vi "3D_Traverse_move.vi"(0 "Mode":T3=enum."Read traverse position", 1 "Route Checking?":bool=TRUE, 2 "Row Number":i32=-1, 5 "Position":dbl[](array[numeric])=[0.0, 0.0, 0.0] format="%#.2f", 7 "Work in Tunnel Coordinates":T1, 11 "Simulate/Run":T2=enum."Run VI", 12 "Traverse name":string, 13 "Backlash Compensation?":bool=TRUE, 14 "Currently on Point":i32=-1) -> (3 "Model  Roll        Pitch       Yaw (deg)":dbl[](array[numeric]) format="%#.2f", 4 "Trav Position achieved":dbl[](array[numeric]) format="%#.2f", 15 "Error String":string)   [LabVIEW 2011]
uses:
  Trav_mode.ctl
  Controls/User_Specific_mode.ctl
  Controls/Tunnel_Coordinates.ctl
  Controls/Global_mode.ctl
  Route mapping/Route_Display_Mode.ctl
  ADAM Client/Sub VIs/ADAM Controls/Update_scan_value.ctl
  Controls/In_Range.ctl
  Globals/Trav_pos_global.vi
  Globals/Constants_global.vi
  Route mapping/Route_mapping_global.vi
panel:
  in  "Position Increment":dbl[](array[numeric])=[0.0, 0.0, 0.0] step=0.1 format="%#.2f"
  out "Traverses Available":string[](array[string])
  in  "Traverse":u16(ring) items=["A_Tunnel", "Aero_Enclosure", "Aero_Sting", "Aero_ThroughWall", "Aero_Tunnel", "Angle_Calibrator", "B_Tunnel", "D_Tunnel", "Dummy_Traverse", "EnFlo_Stack", "EnFlo_Tunnel", "EnFlo_Turntable", "Laser_Meas_Traverse", "Pitch_Yaw", "PIV_Traverse", "Tank"]
  # "X                Y                   Z"
  # "X                Y                   Z"
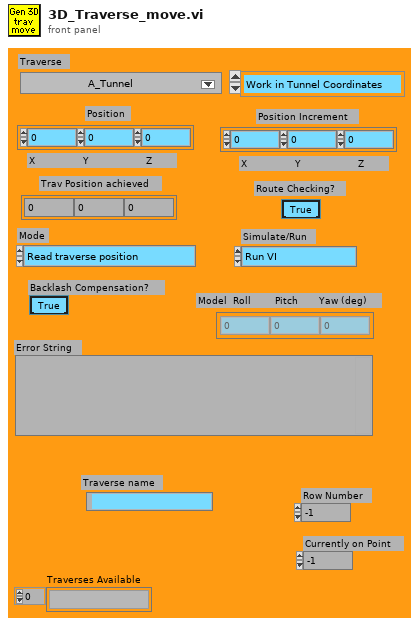
[diagram p1: front panel]
types:
  T1 = typedef "Tunnel_Coordinates.ctl" = enum16{"Work in Tunnel Coordinates", "Work in Model Coordinates"}
  T2 = typedef "User_Specific_mode.ctl" = enum16{"Check VI only", "Run VI"}
  T3 = typedef "Trav_mode.ctl" = enum16{"Move traverse", "Read traverse position", "Teach Position"}
  T4 = typedef "Global_mode.ctl" = enum16{"Read Global", "Load Global From File", "Write Global to File"}
  T5 = enum16{"To Traverse Coordinates", "To User Coordinates"}
  T6 = typedef "Route_Display_Mode.ctl" = enum16{"Display View Always", "Display View on Crash"}
  T7 = typedef "Update_scan_value.ctl" = cluster{"Channel Name":string, "New Value":dbl}
  T8 = typedef "In_Range.ctl" = enum16{"%", "±", "% & ±"}
  T9 = typedef "Box_size.ctl" = cluster{"Max":dbl, "Min":dbl}[]
  T10 = typedef "Exclude_cluster.ctl" = cluster{"Sizes":T9, "Name":string, "Exclude Type":T11}
  T11 = typedef "Exclusion_type.ctl" = enum16{"Exclude completely", "Allow only vertical moves"}
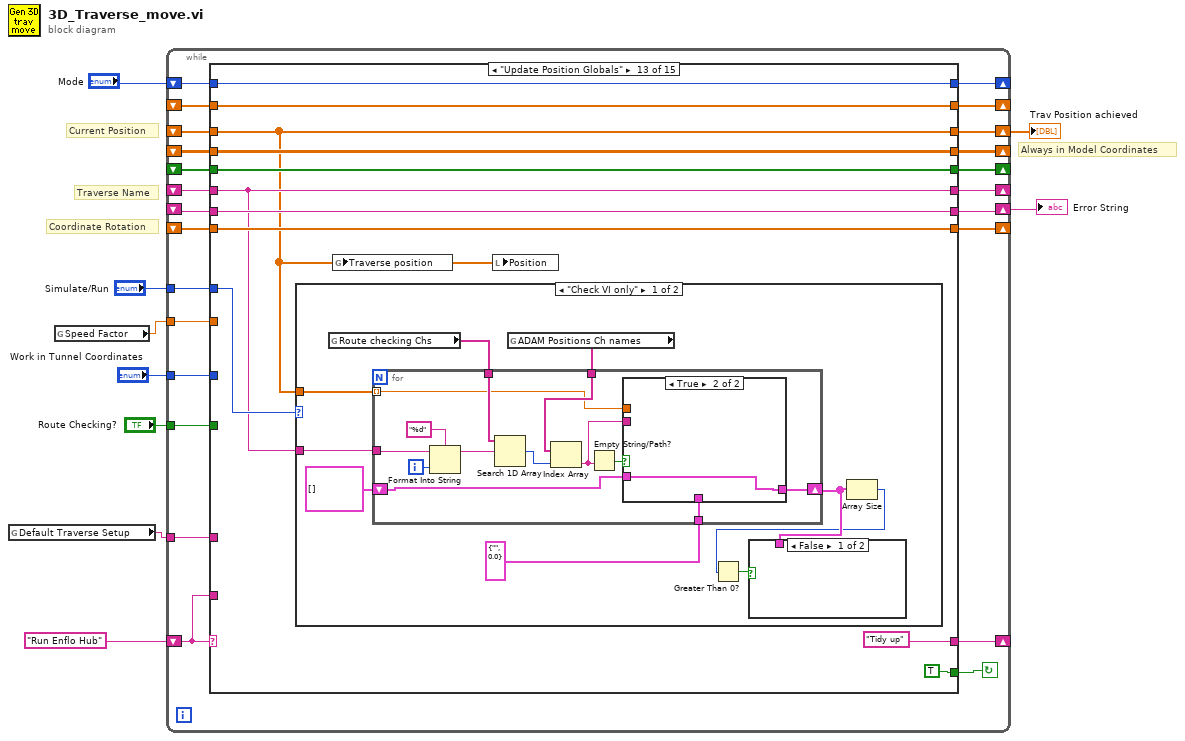
[diagram p0: block diagram]
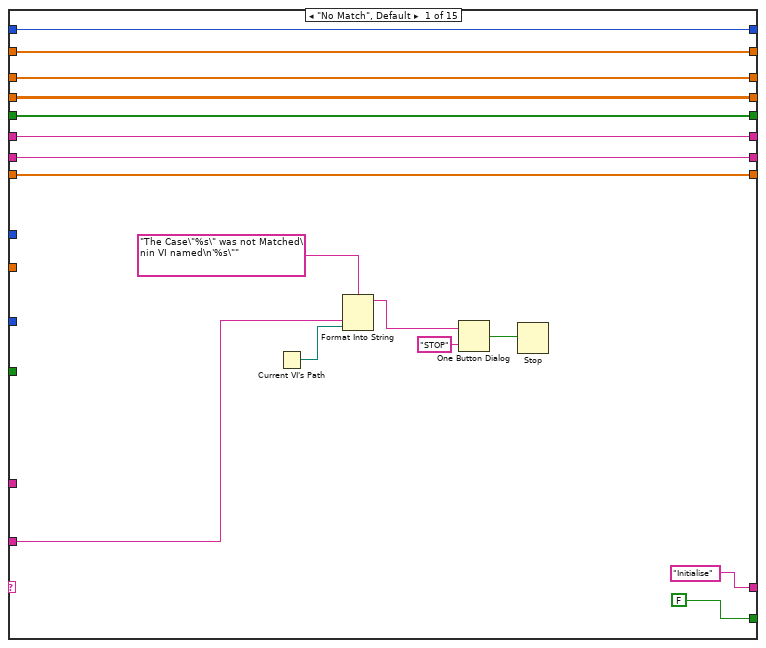
[diagram p2: hidden frame]
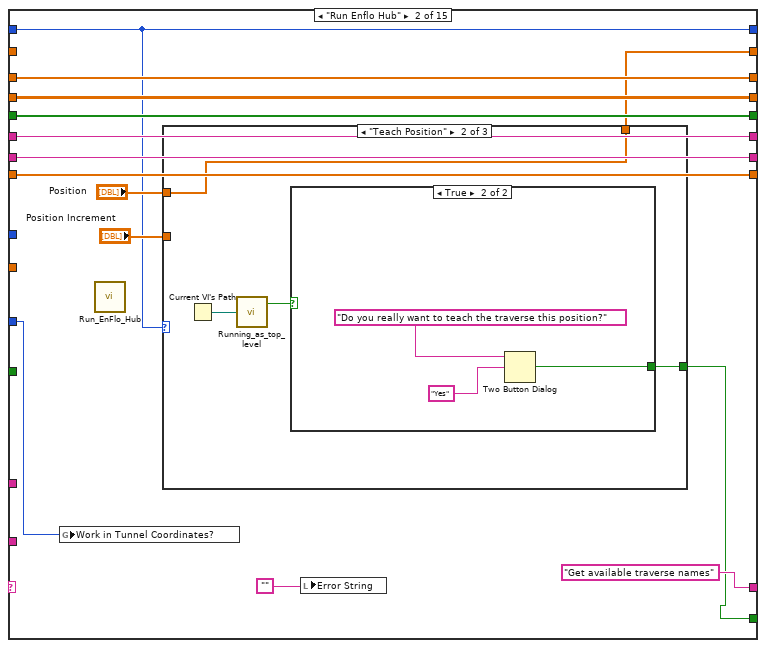
[diagram p3: hidden frame]
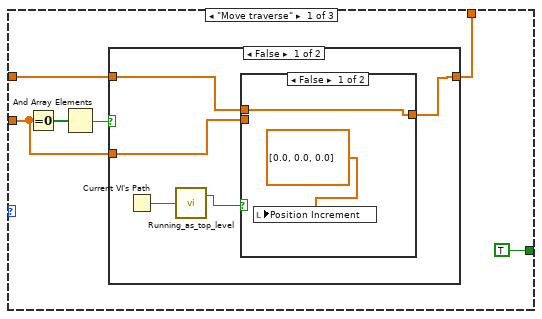
[diagram p4: hidden frame]
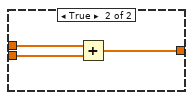
[diagram p5: hidden frame]
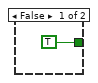
[diagram p7: hidden frame]
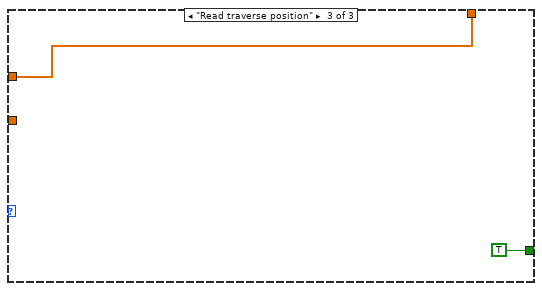
[diagram p8: hidden frame]
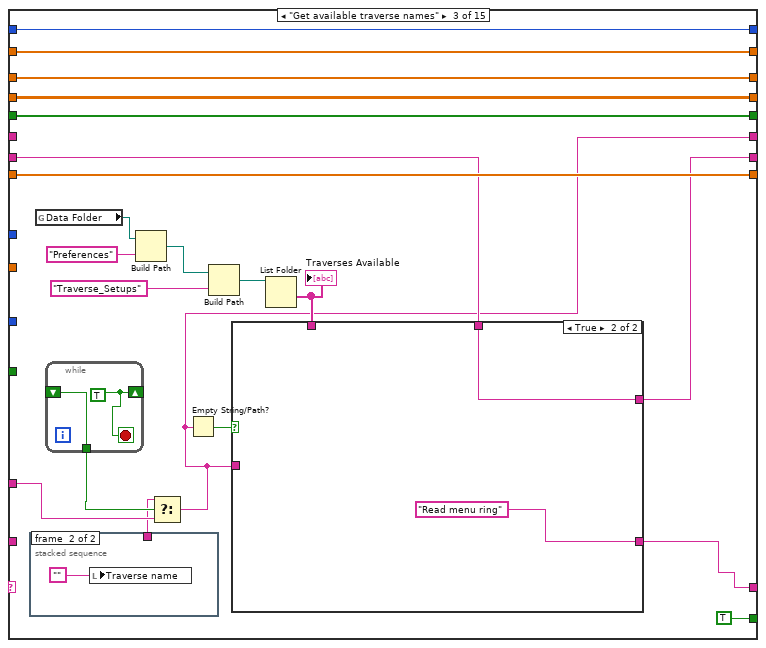
[diagram p9: hidden frame]
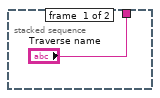
[diagram p10: hidden frame]
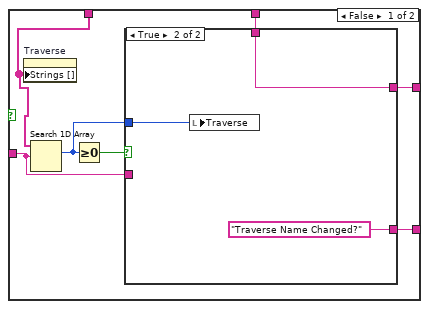
[diagram p11: hidden frame]
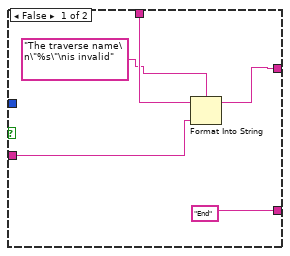
[diagram p12: hidden frame]
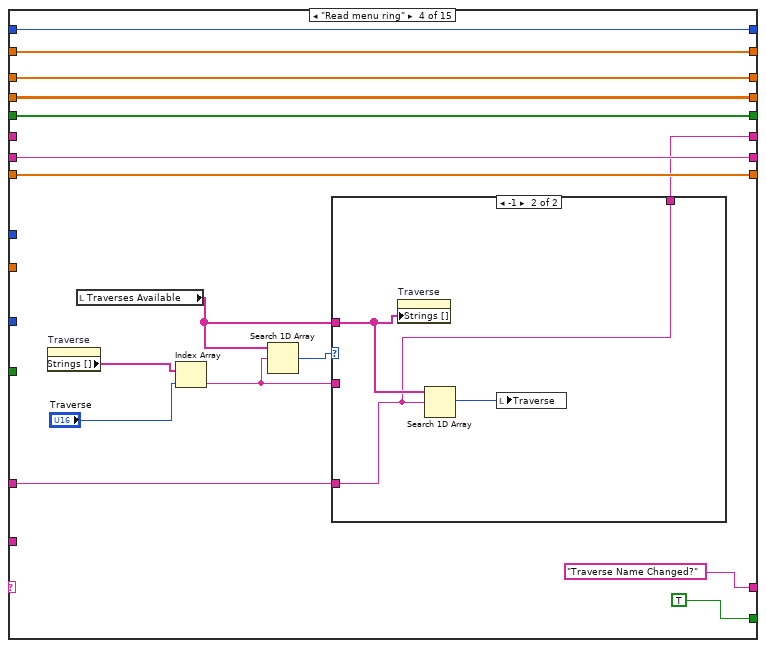
[diagram p13: hidden frame]
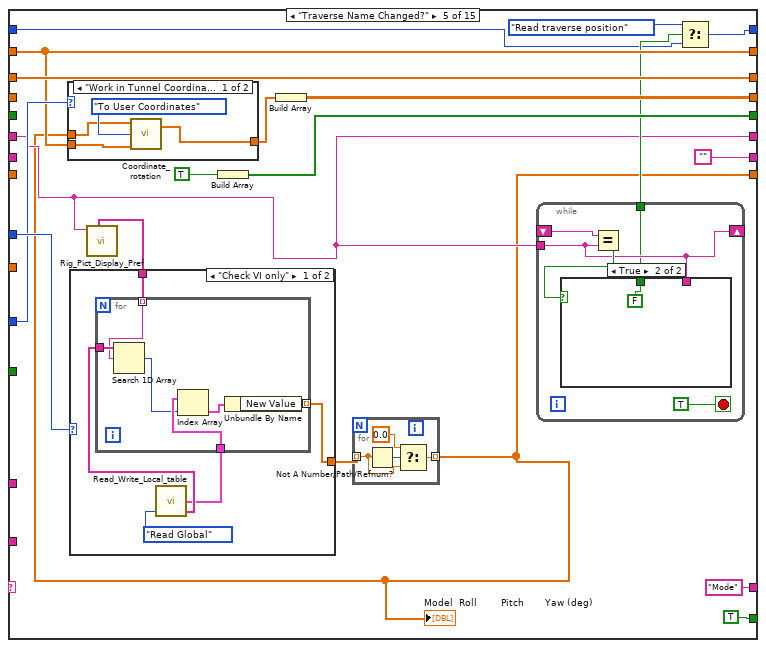
[diagram p15: hidden frame]
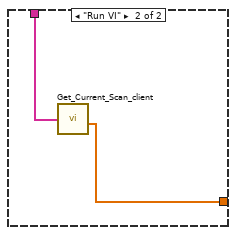
[diagram p16: hidden frame]
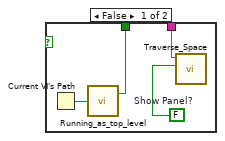
[diagram p18: hidden frame]
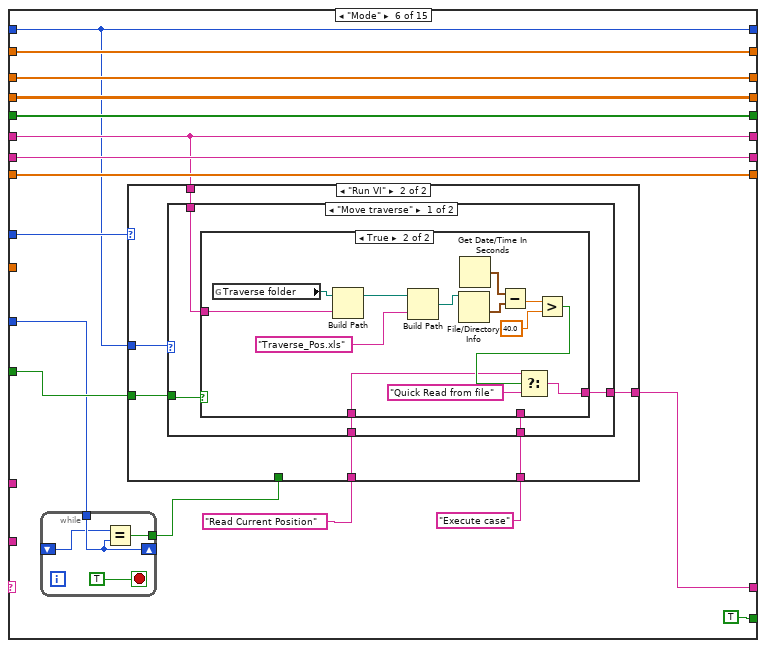
[diagram p19: hidden frame]
diagram:
  # "Always in Model Coordinates"
  # "Current Position"
  # "Coordinate Rotation"
  # "Traverse Name"
  n1 = global read "Trav_pos_global.vi" "Default Traverse Setup"() -> (w2:string)
  n2 = global read "Trav_pos_global.vi" "Speed Factor"() -> (w6:dbl)
  n3 = while {
    shift-left: "Run Enflo Hub" -> [w31]
    shift-right: [w32] -> _
    shift-right: [w29] -> _
    shift-left: _ -> [w27]
    tunnel: "Simulate/Run" -> [w30]
    shift-right: [w28] -> w7
    shift-left: _ -> [w26]
    shift-right: [w24] -> _
    shift-left: _ -> [w25]
    shift-right: [w19] -> _
    shift-left: _ -> [w18]
    shift-right: [w21] -> _
    shift-left: _ -> [w20]
    shift-right: [w22] -> w3
    shift-left: _ -> [w23]
    tunnel: w6 -> [w17]
    tunnel: "Work in Tunnel Coordinates" -> [w16]
    tunnel: "Route Checking?" -> [w15]
    tunnel: w2 -> [w14]
    shift-right: [w13] -> _
    shift-left: _ -> [w12]
    shift-right: [w10] -> _
    shift-left: "Mode" -> [w11]
    stop <- w33 continue-if-true
    n4 = case shown="\"Update Position Globals\"" w31 {
      tunnel: [FALSE w55 TRUE TRUE TRUE TRUE w264 TRUE ("T button?") TRUE w352 w381 TRUE TRUE TRUE FALSE] -> w33
      tunnel: ["Initialise" "Get available traverse names" w101 "Traverse Name Changed?" "Mode" w213 w253 "Perform Route Check" w314 "Display Traverse Views" w388 "Update Position Globals" "Tidy up" "End" "End"] -> w32
      tunnel: w31 -> [w44 _ _ _ _ _ _ _ _ _ _ _ _ _ _]
      tunnel: w30 -> [_ _ _ _ w163 w214 w258 _ w310 _ w386 _ w454 _ w544]
      tunnel: [w41 w62 w94 w133 w156 w205 w266 w290 w309 w358 w393 w429 w453 w496 w540] -> w29
      tunnel: [w40 w61 w99 w146 "" w215 w265 "" w319 w349 w390 w418 w458 w498 w547] -> w28
      tunnel: w27 -> [w41 w62 _ _ w156 w205 w266 w290 w309 w358 w393 w429 w453 w496 w540]
      tunnel: w26 -> [w40 w61 w98 w146 _ w215 _ _ _ w350 w390 _ w458 w499 w547]
      tunnel: w25 -> [w39 w60 w111 w145 _ w216 w262 w293 w305 w345 w397 w425 w457 w502 w541]
      tunnel: [w39 w60 w111 w145 w153 w216 w262 w293 w305 w345 w397 w425 w457 w502 w541] -> w24
      tunnel: w23 -> [w38 w59 w110 w144 w167 w207 w259 _ w317 w357 w396 _ w452 w500 w542]
      tunnel: [w38 w59 w110 w144 w167 w207 w260 w292 w318 w357 w396 w423 w452 w500 w542] -> w22
      tunnel: [w37 w58 w109 w143 w168 w218 w268 w297 w316 w356 w394 w427 w459 w503 w548] -> w21
      tunnel: w20 -> [w37 w58 w109 w143 _ w218 w268 w297 _ w356 w394 w427 w459 w503 w548]
      tunnel: [w36 w57 w108 w142 w165 w217 w267 w296 w321 w355 w395 w421 w460 w504 w549] -> w19
      tunnel: w18 -> [w36 w57 w108 w142 _ w217 w267 w296 _ w355 w395 w421 w460 w504 w549]
      tunnel: w17 -> [_ _ _ _ _ _ _ _ _ _ _ w428 _ _ _]
      tunnel: w16 -> [_ w54 _ _ w162 w209 w263 w294 w327 w346 _ w426 _ _ w543]
      tunnel: w15 -> [_ _ _ _ _ w210 _ _ _ _ _ w417 _ _ _]
      tunnel: w14 -> [_ _ w95 w137 _ _ _ _ _ _ _ _ _ _ _]
      tunnel: [w35 w53 w92 w135 w161 w206 w252 w291 w304 w348 w380 w416 w456 w495 w545] -> w13
      tunnel: w12 -> [w35 _ w92 w135 w161 w206 w252 w291 w304 w348 w380 w416 w456 w495 w545]
      tunnel: w11 -> [w34 w50 w91 w134 w157 w204 w251 w286 w303 w347 w379 w415 w455 w494 w539]
      tunnel: [w34 w50 w91 w134 w158 w204 w251 w286 w303 w347 w379 w415 w455 w494 w539] -> w10
      frame "No Match", Default {
        n5 = Current VI's Path() -> (path=w43:path)
        n6 = Format Into String(format string="The Case\"%s\" was not Matched\nin VI named\n'%s\"" ("Format String"), w44, w43) -> (resulting string=w47:string)  [unwired: 2 in, 1 out]
        n7 = One Button Dialog(message=w47, button name ("OK")="STOP") -> (true=w45:bool)
        n8 = Stop(stop? (T)=w45) -> ()
      }
      frame "Run Enflo Hub" {
        n9 = global write "Trav_pos_global.vi" "Work in Tunnel Coordinates?"(w54) -> ()
        n10 = call "Run_EnFlo_Hub.vi"() -> ()  [unwired: 8 out]
        n11 = case shown="\"Teach Position\"" w50 {
          tunnel: [TRUE ("T button?") w82 TRUE ("T button?")] -> w55
          tunnel: [w66 w81 w90] -> w53
          tunnel: "Position" -> [w65 w81 w90]
          tunnel: "Position Increment" -> [w64 _ _]
          frame "Move traverse" {
            n12 = Equal To 0?(x=w64) -> (x = 0?=w68:bool[])
            n13 = And Array Elements(Boolean array=w68) -> (logical AND=w67:bool)
            n14 = case shown="False" w67 {
              tunnel: [w70 w80] -> w66
              tunnel: w65 -> [w72 w80]
              tunnel: w64 -> [w71 _]
              frame False {
                n15 = Current VI's Path() -> (path=w74:path)
                n16 = call "Running_as_top_level.vi"("Vi path name"=w74) -> ("Top Level"=w73:bool)  [unwired: 1 out]
                n17 = case shown="False" w73 {
                  tunnel: w72 -> [w76 w79]
                  tunnel: w71 -> [_ w78]
                  tunnel: [w76 w77] -> w70
                  frame False {
                    n18 = local write "Position Increment"(dbl[] [0.0, 0.0, 0.0] ("Position Increment")) -> ()
                  }
                  frame True {
                    n19 = Add(x=w79, y=w78) -> (x+y=w77:dbl[])
                  }
                }
              }
              frame True {
              }
            }
          }
          frame "Teach Position" {
            n20 = Current VI's Path() -> (path=w84:path)
            n21 = call "Running_as_top_level.vi"("Vi path name"=w84) -> ("Top Level"=w83:bool)  [unwired: 1 out]
            n22 = case shown="True" w83 {
              tunnel: [TRUE ("T button?") w86] -> w82
              frame False {
              }
              frame True {
                n23 = Two Button Dialog(message="Do you really want to teach the traverse this position?", 2:"Yes" ("T button name (\"OK\")")) -> (T button?=w86:bool)  [unwired: 1 out]
              }
            }
          }
          frame "Read traverse position" {
          }
        }
        n24 = local write "Error String"("") -> ()
      }
      frame "Get available traverse names" {
        n25 = stacked-sequence {
          tunnel: ["Traverse name" _] -> w93
          frame #0 {
          }
          frame #1 {
            n26 = local write "Traverse name"("") -> ()
          }
        }
        n27 = global read "Constants_global.vi" "Data Folder"() -> (w104:path)
        n28 = while {
          shift-right: [w114] -> _
          shift-left: _ -> [w115]
          tunnel: [w115] -> w96
          stop <- w114 stop-if-true
          w114 = TRUE
        }
        n29 = Build Path(base path=w104, name or relative path="Preferences") -> (appended path=w106:path)
        n30 = Select(t=w93, s=w96, f=w95) -> (s? t:f=w94:string)
        n31 = Empty String/Path?(string/path=w94) -> (empty?=w102:bool)
        n32 = Build Path(base path=w106, name or relative path="Traverse_Setups") -> (appended path=w107:path)
        n33 = List Folder(path=w107) -> (folder names=w100:string[])  [unwired: 1 in, 5 out]
        "Traverses Available" <- w100
        n34 = case shown="True" w102 {
          tunnel: [w119 "Read menu ring"] -> w101
          tunnel: w100 -> [w116 _]
          tunnel: w94 -> [w122 _]
          tunnel: [w121 w131] -> w99
          tunnel: w98 -> [w120 w131]
          frame False {
            n35 = property on="Traverse" class="Ring (strict)"("Strings []"=w116) -> ()  [unwired: 2 in, 2 out]
            n36 = Search 1D Array(1D array=w116, element=w122) -> (index of element=w117:i32)  [unwired: 1 out]
            n37 = Greater Or Equal To 0?(x=w117) -> (x >= 0?=w118:bool)
            n38 = case shown="True" w118 {
              tunnel: w122 -> [w127 _]
              tunnel: [w124 w130] -> w121
              tunnel: w120 -> [w126 w130]
              tunnel: ["End" "Traverse Name Changed?"] -> w119
              tunnel: w117 -> [_ w128]
              frame False {
                n39 = Format Into String(format string="The traverse name\n\"%s\"\nis invalid", initial string=w126, w127) -> (resulting string=w124:string)  [unwired: 1 in, 1 out]
              }
              frame True {
                n40 = local write "Traverse"(w128) -> ()
              }
            }
          }
          frame True {
          }
        }
      }
      frame "Read menu ring" {
        n41 = property on="Traverse" class="Ring (strict)"() -> ("Strings []"=w141:string[])  [unwired: 2 in, 2 out]
        n42 = local read "Traverses Available"() -> (w138:string[])
        n43 = Index Array(array=w141, index="Traverse") -> (element=w136:string)
        n44 = Search 1D Array(1D array=w138, element=w136) -> (index of element=w139:i32)  [unwired: 1 out]
        n45 = case shown="-1" w139 {
          tunnel: w138 -> [_ w152]
          tunnel: w137 -> [_ w150]
          tunnel: [w149 w150] -> w133
          tunnel: w136 -> [w149 _]
          frame 0, Default {
          }
          frame -1 {
            n46 = property on="Traverse" class="Ring (strict)"("Strings []"=w152) -> ()  [unwired: 2 in, 2 out]
            n47 = Search 1D Array(1D array=w152, element=w150) -> (index of element=w151:i32)  [unwired: 1 out]
            n48 = local write "Traverse"(w151) -> ()
          }
        }
      }
      frame "Traverse Name Changed?" {
        n49 = call "Rig_Pict_Display_Pref.vi"("Traverse Name"=w156) -> ("Roll Pitch Yaw ADAM Channels"=w155:string[])  [unwired: 3 in, 4 out]
        n50 = case shown="\"Check VI only\"" w163 {
          tunnel: [w176 w187] -> w154
          tunnel: w155 -> [w178 w188]
          frame "Check VI only" {
            n51 = call "Read_Write_Local_table.vi"("Mode"=Global_mode."Read Global") -> ("Ch Names"=w179:string[], "Ch Values Out"=w177:T7[])  [unwired: 2 in, 1 out]
            n52 = for {
              tunnel: w179 -> [w186]
              tunnel: w178 -> [w185] mode=indexing
              tunnel: w177 -> [w184]
              tunnel: [w181] -> w176 mode=indexing
              n53 = Search 1D Array(1D array=w186, element=w185) -> (index of element=w183:i32)  [unwired: 1 out]
              n54 = Index Array(array=w184, index=w183) -> (element=w182:T7)
              n55 = Unbundle By Name(w182) -> ("New Value"=w181:dbl)
            }
          }
          frame "Run VI" {
            n56 = call "Get_Current_Scan_client.vi"("ADAM Ch Names"=w188) -> ("Numerical Values"=w187:dbl[])  [unwired: 3 out]
          }
        }
        n57 = Build Array(TRUE) -> (w165:bool[])
        n58 = for {
          tunnel: w154 -> [w174] mode=indexing
          tunnel: [w172] -> w153 mode=indexing
          n59 = Not A Number/Path/Refnum?(number/path/refnum=w174) -> (NaN/Path/Refnum?=w175:bool)
          n60 = Select(t=0.0, s=w175, f=w174) -> (s? t:f=w172:dbl)
        }
        "Model  Roll        Pitch       Yaw (deg)" <- w153
        n61 = case shown="\"Work in Tunnel Coordinates\"" w162 {
          tunnel: w161 -> [w191 w193]
          tunnel: [w190 w193] -> w164
          tunnel: w153 -> [w189 _]
          frame "Work in Tunnel Coordinates" {
            n62 = call "Coordinate_rotation.vi"("Model       Roll      Pitch       Yaw (deg)"=w189, "Input Position"=w191, "Mode"=T5."To User Coordinates") -> ("Output Position"=w190:dbl[])  [unwired: 2 in, 1 out]
          }
          frame "Work in Model Coordinates" {
          }
        }
        n63 = Build Array(w164) -> (w168:dbl[][])
        n64 = while {
          shift-right: [w195] -> _
          shift-left: _ -> [w197]
          tunnel: w156 -> [w195]
          tunnel: [w194] -> w160
          stop <- TRUE stop-if-true
          n65 = Equal?(x=w197, y=w195) -> (x = y?=w196:bool)
          n66 = case shown="True" w196 {
            tunnel: w195 -> [w201 _]
            tunnel: [w199 FALSE ("Top Level")] -> w194
            frame False {
              w202 = FALSE  # Show Panel?
              n67 = Current VI's Path() -> (path=w200:path)
              n68 = call "Running_as_top_level.vi"("Vi path name"=w200) -> ("Top Level"=w199:bool)  [unwired: 1 out]
              n69 = call "Traverse_Space.vi"("Show Panel?"=w202, "Traverse Setup"=w201) -> ()  [unwired: 1 in, 8 out]
            }
            frame True {
            }
          }
        }
        n70 = Select(t=Trav_mode."Read traverse position" ("Mode"), s=w160, f=w157) -> (s? t:f=w158:T3)
      }
      frame "Mode" {
        n71 = while {
          shift-right: [w222] -> _
          shift-left: _ -> [w221]
          tunnel: w209 -> [w222]
          tunnel: [w220] -> w208
          stop <- TRUE stop-if-true
          n72 = Equal?(x=w221, y=w222) -> (x = y?=w220:bool)
        }
        n73 = case shown="\"Run VI\"" w214 {
          tunnel: w204 -> [_ w230]
          tunnel: [w224 w229] -> w213
          tunnel: "Execute case" -> [_ w228]
          tunnel: "Read Current Position" -> [w224 w227]
          tunnel: w210 -> [_ w226]
          tunnel: w208 -> [_ _]
          tunnel: w205 -> [_ w225]
          frame "Check VI only" {
          }
          frame "Run VI" {
            n74 = case shown="\"Move traverse\"" w230 {
              tunnel: [w233 w250] -> w229
              tunnel: w228 -> [w232 w250]
              tunnel: w227 -> [w231 _]
              tunnel: w226 -> [w234 _]
              tunnel: w225 -> [w235 _]
              frame "Move traverse" {
                n75 = case shown="True" w234 {
                  tunnel: w235 -> [_ w246]
                  tunnel: [w236 w240] -> w233
                  tunnel: w232 -> [w236 _]
                  tunnel: w231 -> [_ w238]
                  frame False {
                  }
                  frame True {
                    n76 = global read "Constants_global.vi" "Traverse folder"() -> (w247:path)
                    n77 = Build Path(base path=w247, name or relative path=w246) -> (appended path=w249:path)
                    n78 = Build Path(base path=w249, name or relative path="Traverse_Pos.xls" ("Substring")) -> (appended path=w245:path)
                    n79 = File/Directory Info(path=w245) -> (last mod=w243:timestamp)  [unwired: 1 in, 6 out]
                    n80 = Get Date/Time In Seconds() -> (seconds since 1Jan1904=w244:timestamp)
                    n81 = Subtract(x=w244, y=w243) -> (x-y=w242:dbl)
                    n82 = Greater?(x=w242, y=40.0) -> (0:w239:bool)
                    n83 = Select(t=w238, s=w239, f="Quick Read from file") -> (s? t:f=w240:string)
                  }
                }
              }
              frame "Read traverse position", Default {
              }
            }
          }
        }
      }
      frame "Read Current Position" {
        n84 = case shown="\"Run VI\"" w258 {
          tunnel: w266 -> [w269 w278]
          tunnel: ["" w280] -> w265
          tunnel: w262 -> [_ w273]
          tunnel: [w270 w279] -> w261
          tunnel: w259 -> [_ w275]
          frame "Check VI only" {
            n85 = call "Read-Write_Check_Pos.vi"("Mode"=enum16{"Read", "Write"}."Read", "Traverse Name"=w269) -> ("Position Output"=w270:dbl[])  [unwired: 1 in]
          }
          frame "Run VI" {
            w277 = FALSE  # Route Checking?
            w276 = FALSE  # Backlash Compensation?
            n86 = call "TraverseControl.vi"("Mode"=Trav_mode."Read traverse position", "Route Checking?"=w277, "Traverse Name"=w278, "Model       Roll      Pitch       Yaw (deg)"=w273, "Position input XYZ"=w275, "Backlash Compensation?"=w276) -> ("Position Output XYZ"=w279:dbl[], "Error String"=w280:string)  [unwired: 2 in, 6 out]
          }
        }
        n87 = Equal?(x=Trav_mode."Read traverse position" ("Mode"), y=w251) -> (x = y?=w256:bool)
        n88 = case shown="\"Work in Model Coordinates\"" w263 {
          tunnel: w261 -> [w281 w283]
          tunnel: [w281 w284] -> w260
          tunnel: w262 -> [_ w282]
          frame "Work in Tunnel Coordinates" {
          }
          frame "Work in Model Coordinates" {
            n89 = call "Coordinate_rotation.vi"("Model       Roll      Pitch       Yaw (deg)"=w282, "Input Position"=w283, "Mode"=T5."To User Coordinates") -> ("Output Position"=w284:dbl[])  [unwired: 2 in, 1 out]
          }
        }
        n90 = Empty String/Path?(string/path=w265) -> (empty?=w264:bool)
        n91 = Select(t="Update Position Globals", s=w256, f="Perform Route Check") -> (s? t:f=w253:string)
      }
      frame "Quick Read from file" {
        n92 = call "Read_Traverse_Pos_File.vi"("Traverse Name"=w290) -> ("Tunnel Coordinates"=w289:dbl[])
        n93 = case shown="\"Work in Model Coordinates\"" w294 {
          tunnel: w289 -> [w298 w301]
          tunnel: [w298 w300] -> w292
          tunnel: w293 -> [_ w299]
          frame "Work in Tunnel Coordinates" {
          }
          frame "Work in Model Coordinates" {
            n94 = call "Coordinate_rotation.vi"("Model       Roll      Pitch       Yaw (deg)"=w299, "Input Position"=w301, "Mode"=T5."To User Coordinates") -> ("Output Position"=w300:dbl[])  [unwired: 2 in, 1 out]
          }
        }
      }
      frame "Perform Route Check" {
        n95 = case shown="\"Work in Tunnel Coordinates\"" w327 {
          tunnel: w305 -> [w341 _]
          tunnel: w304 -> [w337 w343]
          tunnel: w317 -> [w340 w344]
          tunnel: [w339 w343] -> w308
          tunnel: [w338 w344] -> w320
          frame "Work in Tunnel Coordinates" {
            w342 = T5."To User Coordinates" ("Mode")
            n96 = call "Coordinate_rotation.vi"("Model       Roll      Pitch       Yaw (deg)"=w341, "Input Position"=w340, "Mode"=w342) -> ("Output Position"=w338:dbl[])  [unwired: 2 in, 1 out]
            n97 = call "Coordinate_rotation.vi"("Model       Roll      Pitch       Yaw (deg)"=w341, "Input Position"=w337, "Mode"=w342) -> ("Output Position"=w339:dbl[])  [unwired: 2 in, 1 out]
          }
          frame "Work in Model Coordinates" {
          }
        }
        n98 = global read "Route_mapping_global.vi" "Entire Space"() -> (w326:T9)
        n99 = global read "Route_mapping_global.vi" "Exclude Array"() -> (w324:T10[])
        n100 = global read "Route_mapping_global.vi" "Probe Volume"() -> (w325:T9)
        n101 = call "Check_with_Jump.vi"("Model       Roll      Pitch       Yaw (deg)"=w305, "Simulate/Run"=w310, "Exclude Array"=w324, "Traverse Name"=w309, "Probe Volume"=w325, "Entire Space"=w326, "New Position"=w308, "Current position"=w320) -> ("Steps"=w316:dbl[][], "Error Comments"=w319:string)  [unwired: 2 out]
        n102 = Array Size(array=w316) -> (size(s)=w323:i32[])
        n103 = Empty String/Path?(string/path=w319) -> (empty?=w311:bool)
        n104 = case shown="False" w311 {
          tunnel: [w335 w336] -> w318
          tunnel: w317 -> [w335 _]
          tunnel: w304 -> [_ w336]
          frame False {
          }
          frame True {
          }
        }
        n105 = Index Array(array=w323, index=0) -> (element=w306:i32)
        n106 = case shown="3, Default" w306 {
          tunnel: [w329 w331 w334] -> w321
          tunnel: "Backlash Compensation?" -> [w328 w330 w332]
          frame 1 {
            n107 = Build Array(w328) -> (w329:bool[])
          }
          frame 2 {
            n108 = Build Array(w330, w330) -> (w331:bool[])
          }
          frame 3, Default {
            n109 = Build Array(FALSE, w332, w332) -> (w334:bool[])
          }
        }
        n110 = Select(t="Display Traverse Views", s=w311, f="Route Error") -> (s? t:f=w314:string)
      }
      frame "Route Error" {
        n111 = global read "Trav_pos_global.vi" "Jump Bad Positions?"() -> (w354:bool)
        n112 = case shown="True" w354 {
          tunnel: w348 -> [_ w363]
          tunnel: [TRUE w362] -> w352
          tunnel: w346 -> [_ w361]
          tunnel: w345 -> [_ w360]
          frame False {
          }
          frame True {
            n113 = Current VI's Path() -> (path=w365:path)
            n114 = call "Running_as_top_level.vi"("Vi path name"=w365) -> ("Top Level"=w364:bool)  [unwired: 1 out]
            n115 = case shown="False" w364 {
              tunnel: w363 -> [w367 _]
              tunnel: [FALSE TRUE] -> w362
              tunnel: w361 -> [w369 _]
              tunnel: w360 -> [w366 _]
              frame False {
                n116 = case shown="\"Work in Tunnel Coordinates\"" w369 {
                  tunnel: [w374 w377] -> w368
                  tunnel: w367 -> [w375 w377]
                  tunnel: w366 -> [w373 _]
                  frame "Work in Tunnel Coordinates" {
                    n117 = call "Coordinate_rotation.vi"("Model       Roll      Pitch       Yaw (deg)"=w373, "Input Position"=w375, "Mode"=T5."To User Coordinates") -> ("Output Position"=w374:dbl[])  [unwired: 2 in, 1 out]
                  }
                  frame "Work in Model Coordinates" {
                  }
                }
                n118 = global read "Trav_pos_global.vi" "Jumped Positions"() -> (w371:dbl[][])
                n119 = Build Array (concatenate)(w368, w371) -> (w370:dbl[][])
                n120 = global write "Trav_pos_global.vi" "Jumped Positions"(w370) -> ()
              }
              frame True {
              }
            }
          }
        }
        n121 = Concatenate Strings("Route Checking Error\n" ("string"), w350) -> (w349:string)
      }
      frame "Display Traverse Views" {
        n122 = global read "Route_mapping_global.vi" "Display Mode"() -> (w392:T6)
        n123 = Equal?(x=w386, y=User_Specific_mode."Check VI only" ("Simulate/Run")) -> (x = y?=w385:bool)
        n124 = Empty String/Path?(string/path=w390) -> (empty?=w381:bool)
        n125 = Equal?(x=w392, y=Route_Display_Mode."Display View Always" ("Display Mode")) -> (x = y?=w389:bool)
        n126 = Not(x=w381) -> (.not. x?=w382:bool)
        n127 = Or(x=w389, y=w382) -> (x .or. y?=w384:bool)
        n128 = And(x=w385, y=w384) -> (x .and. y?=w383:bool)
        n129 = case shown="True" w383 {
          tunnel: w394 -> [_ w406]
          tunnel: w393 -> [_ w405]
          tunnel: w390 -> [_ w402]
          tunnel: w381 -> [_ w400]
          frame False {
          }
          frame True {
            n130 = Not(x=w400) -> (.not. x?=w401:bool)
            n131 = for {
              tunnel: w406 -> [w413] mode=indexing
              tunnel: w405 -> [w412]
              tunnel: "Currently on Point" -> [w411]
              tunnel: "Row Number" -> [w410]
              tunnel: w402 -> [w409]
              tunnel: w401 -> [w407]
              n132 = Build Array(w413) -> (w414:dbl[][])
              n133 = call "Display_Trav_Views.vi"("Current Probe Position"=w414, "Traverse Name"=w412, "Currently on point"=w411, "Open Front Panel"=TRUE, "Error Comments"=w409, "Crash?"=w407, "Row Number"=w410) -> ()  [unwired: 4 out]
            }
          }
        }
        n134 = case shown="\"Check VI only\"" w386 {
          tunnel: ["Update Position Globals" "Execute case"] -> w388
          frame "Check VI only" {
          }
          frame "Run VI" {
          }
        }
      }
      frame "Execute case" {
        n135 = Array Size(array=w421) -> (size(s)=w420:i32)
        n136 = Decrement(x=w420) -> (x-1=w419:i32)
        n137 = while {
          tunnel: w429 -> [w435]
          tunnel: w427 -> [w446] mode=indexing
          tunnel: w428 -> [w434]
          tunnel: w415 -> [w437]
          tunnel: w425 -> [w431]
          tunnel: [w439] -> w424
          tunnel: w421 -> [w433] mode=indexing
          tunnel: w419 -> [w443]
          tunnel: [w432] -> w418
          tunnel: w417 -> [w436]
          i -> [w444]
          stop <- w440 continue-if-true
          n138 = call "Coordinate_rotation.vi"("Model       Roll      Pitch       Yaw (deg)"=w431, "Input Position"=w446, "Mode"=T5."To Traverse Coordinates") -> ("Output Position"=w438:dbl[])  [unwired: 2 in, 1 out]
          n139 = Less?(x=w444, y=w443) -> (x < y?=w442:bool)
          n140 = call "TraverseControl.vi"("Mode"=w437, "Route Checking?"=w436, "Traverse Name"=w435, "Model       Roll      Pitch       Yaw (deg)"=w431, "Position input XYZ"=w438, "Speed Factor"=w434, "Backlash Compensation?"=w433) -> ("Position Output XYZ"=w439:dbl[], "Error String"=w432:string)  [unwired: 1 in, 6 out]
          n141 = Empty String/Path?(string/path=w432) -> (empty?=w441:bool)
          n142 = And(x=w441, y=w442) -> (x .and. y?=w440:bool)
        }
        n143 = case shown="\"Work in Model Coordinates\"" w426 {
          tunnel: w424 -> [w447 w450]
          tunnel: [w447 w449] -> w423
          tunnel: w425 -> [_ w448]
          frame "Work in Tunnel Coordinates" {
          }
          frame "Work in Model Coordinates" {
            n144 = call "Coordinate_rotation.vi"("Model       Roll      Pitch       Yaw (deg)"=w448, "Input Position"=w450, "Mode"=T5."To User Coordinates") -> ("Output Position"=w449:dbl[])  [unwired: 2 in, 1 out]
          }
        }
      }
      frame "Update Position Globals" {
        n145 = case shown="\"Check VI only\"" w454 {
          tunnel: w453 -> [w471 _]
          tunnel: w452 -> [w467 _]
          frame "Check VI only" {
            n146 = global read "Trav_pos_global.vi" "Route checking Chs"() -> (w470:string[])
            n147 = global read "Trav_pos_global.vi" "ADAM Positions Ch names"() -> (w469:string[])
            n148 = for {
              tunnel: w471 -> [w484]
              tunnel: w470 -> [w483]
              tunnel: w469 -> [w480]
              tunnel: T7 {"Channel Name"="", "New Value"=0.0} ("Update Scan Value Cluster") -> [w479]
              tunnel: w467 -> [w478] mode=indexing
              shift-right: [w474] -> w465
              shift-left: T7[] [] -> [w475]
              i -> [w486]
              n149 = Format Into String(format string="%d", initial string=w484, w486) -> (resulting string=w482:string)  [unwired: 1 in, 1 out]
              n150 = Search 1D Array(1D array=w483, element=w482) -> (index of element=w481:i32)  [unwired: 1 in]
              n151 = Index Array(array=w480, index=w481) -> (element=w477:string)
              n152 = Empty String/Path?(string/path=w477) -> (empty?=w476:bool)
              n153 = case shown="True" w476 {
                tunnel: w479 -> [w492 _]
                tunnel: w477 -> [w491 _]
                tunnel: w478 -> [w490 _]
                tunnel: w475 -> [w489 w493]
                tunnel: [w488 w493] -> w474
                frame False {
                  n154 = Bundle By Name(cluster=w492, "Channel Name"=w491, "New Value"=w490) -> (w487:T7)
                  n155 = Build Array (concatenate)(w489, w487) -> (w488:T7[])
                }
                frame True {
                }
              }
            }
            n156 = Array Size(array=w465) -> (size(s)=w463:i32)
            n157 = Greater Than 0?(x=w463) -> (x > 0?=w464:bool)
            n158 = case shown="False" w464 {
              tunnel: w465 -> [_ w472]
              frame False {
              }
              frame True {
                n159 = call "Read_Write_Local_table.vi"("Mode"=Global_mode."Write Global to File", "Ch Values in"=w472) -> ()  [unwired: 1 in, 3 out]
              }
            }
          }
          frame "Run VI" {
          }
        }
        n160 = global write "Trav_pos_global.vi" "Traverse position"(w452) -> ()
        n161 = local write "Position"(w452) -> ()
      }
      frame "Tidy up" {
        n162 = case shown="\"Read traverse position\", Default" w494 {
          tunnel: w500 -> [w509 w538]
          tunnel: w499 -> [w510 w537]
          tunnel: w495 -> [w508 _]
          tunnel: [w507 w537] -> w498
          frame "Move traverse" {
            n163 = Empty String/Path?(string/path=w510) -> (empty?=w511:bool)
            n164 = case shown="True" w511 {
              tunnel: w509 -> [_ w516]
              tunnel: w508 -> [_ w515]
              tunnel: w510 -> [w512 w514]
              tunnel: [w512 w513] -> w507
              frame False {
              }
              frame True {
                n165 = for {
                  tunnel: w516 -> [w519] mode=indexing
                  tunnel: w515 -> [w520] mode=indexing
                  shift-right: [w517] -> w513
                  shift-left: w514 -> [w518]
                  i -> [w523]
                  w525 = 10.0  # ±
                  n166 = case shown="0, Default" w523 {
                    tunnel: ["X" "Y" "Z"] -> w521
                    frame 0, Default {
                    }
                    frame 1 {
                    }
                    frame 2 {
                    }
                  }
                  n167 = call "In_Range_check.vi"("±"=w525, "Mode"=In_Range."±", "Value"=w520, "Setpoint"=w519) -> ("In Range"=w522:bool)  [unwired: 1 in, 2 out]
                  n168 = case shown="False" w522 {
                    tunnel: w521 -> [w532 _]
                    tunnel: w520 -> [w531 _]
                    tunnel: w519 -> [w530 _]
                    tunnel: w518 -> [w527 w533]
                    tunnel: [w528 w533] -> w517
                    frame False {
                      n169 = Format Into String(format string="For %s Axis Dem Pos = %.1f Achieved Pos = %.1f mm" ("Format String"), w532, w531, w530) -> (resulting string=w526:string)  [unwired: 2 in, 1 out]
                      n170 = Concatenate Strings(w527, w526) -> (w528:string)
                    }
                    frame True {
                    }
                  }
                }
              }
            }
          }
          frame "Read traverse position", Default {
            n171 = local write "Position"(w538) -> ()
          }
        }
        n172 = local write "Currently on Point"(-1 ("Row Number")) -> ()
        n173 = local write "Simulate/Run"(User_Specific_mode."Run VI" ("Simulate/Run")) -> ()
      }
      frame "End" {
        n174 = case shown="\"Run VI\"" w544 {
          tunnel: w543 -> [_ w557]
          tunnel: w542 -> [_ w554]
          tunnel: w541 -> [_ w553]
          tunnel: w540 -> [_ w552]
          frame "Check VI only", Default {
          }
          frame "Run VI" {
            n175 = case shown="\"Work in Model Coordinates\"" w557 {
              tunnel: w554 -> [w558 w561]
              tunnel: [w558 w560] -> w555
              tunnel: w553 -> [_ w559]
              frame "Work in Tunnel Coordinates" {
              }
              frame "Work in Model Coordinates" {
                n176 = call "Coordinate_rotation.vi"("Model       Roll      Pitch       Yaw (deg)"=w559, "Input Position"=w561, "Mode"=T5."To Traverse Coordinates") -> ("Output Position"=w560:dbl[])  [unwired: 2 in, 1 out]
              }
            }
            n177 = call "Read-Write_Check_Pos.vi"("Position input"=w555, "Mode"=enum16{"Read", "Write"}."Write", "Traverse Name"=w552) -> ()  [unwired: 1 out]
          }
        }
        n178 = case shown="\"Teach Position\"" w539 {
          frame "Move traverse", Default {
          }
          frame "Teach Position" {
            n179 = local write "Mode"(Trav_mode."Read traverse position" ("Mode")) -> ()
          }
        }
        n180 = local write "Route Checking?"(TRUE ("Route Checking?")) -> ()
      }
    }
  }
  "Trav Position achieved" <- w3
  "Error String" <- w7
